vi "Graph ERD Read List_Brass.vi"(0 "GEA2 Reference In":refnum<k24>, 5 "GEA Inputs":T8={"Source"=229, "Destination"=50} {"Destination" format="%.0x"; "Source" format="%.0x"}, 7 "All_Bundled_Data_Brass":T1, 9 "ERD Graph Cntrl":T9={"ERD 3"={"ERD #"=0, "Data Type"=enum."uint16_t", "Scaler"=1}, "ERD 2"={"ERD #"=0, "Data Type"=enum."uint16_t", "Scaler"=1}, "ERD 1"={"ERD #"=0, "Data Type"=enum."uint16_t", "Scaler"=1}} {"ERD 1"."Scaler" min=1; "ERD 1"."ERD #" format="%.0x"; "ERD 2"."Scaler" min=1; "ERD 2"."ERD #" format="%.0x"; "ERD 3"."Scaler" min=1; "ERD 3"."ERD #" format="%.0x"}, 11 "Error In":errorcluster) -> (4 "GEA2 Reference Out":refnum<k24>, 6 "ERD Graph  Ind":T7, 10 "All_Bundled_Data_Brass 2":T1, 15 "Error Out":errorcluster)   [LabVIEW 2016]
uses:
  Laundry Tool 1.0 Support/type defs/ERD_Graph_All.ctl
  Laundry Tool 1.0 Support/type defs/ERD_Graph.ctl
  Common/LabVIEW GEA2 Toolkit/LabVIEW_GEA2_Toolkit.lvlibp/type defs/Data Type.ctl
  C:/Automation/DLLs/PC Dot Net/GeaCommunication.dll
  Common/LabVIEW GEA2 Toolkit/LabVIEW_GEA2_Toolkit.lvlibp/type defs/Source_Destination.ctl
  type defs2/All_Bundled_Data_Brass.ctl
  Laundry Tool 1.0 Support/type defs/Version.ctl
  type defs2/ERD_Always_Show_Brass.ctl
  type defs2/CSV_File_String_Arrays.ctl
  type defs2/Fault Table Array.ctl
  Laundry Tool 1.0 Support/type defs/Fault_Table_Info.ctl
  Common/LabVIEW GEA2 Toolkit/LabVIEW_GEA2_Toolkit.lvlibp/type defs/ERD Read Data In.ctl
  Common/LabVIEW GEA2 Toolkit/LabVIEW_GEA2_Toolkit.lvlibp
panel:
  # "Software Version"
  # "UI"
  # "MC"
  # "Software Version"
  # "UI"
  # "MC"
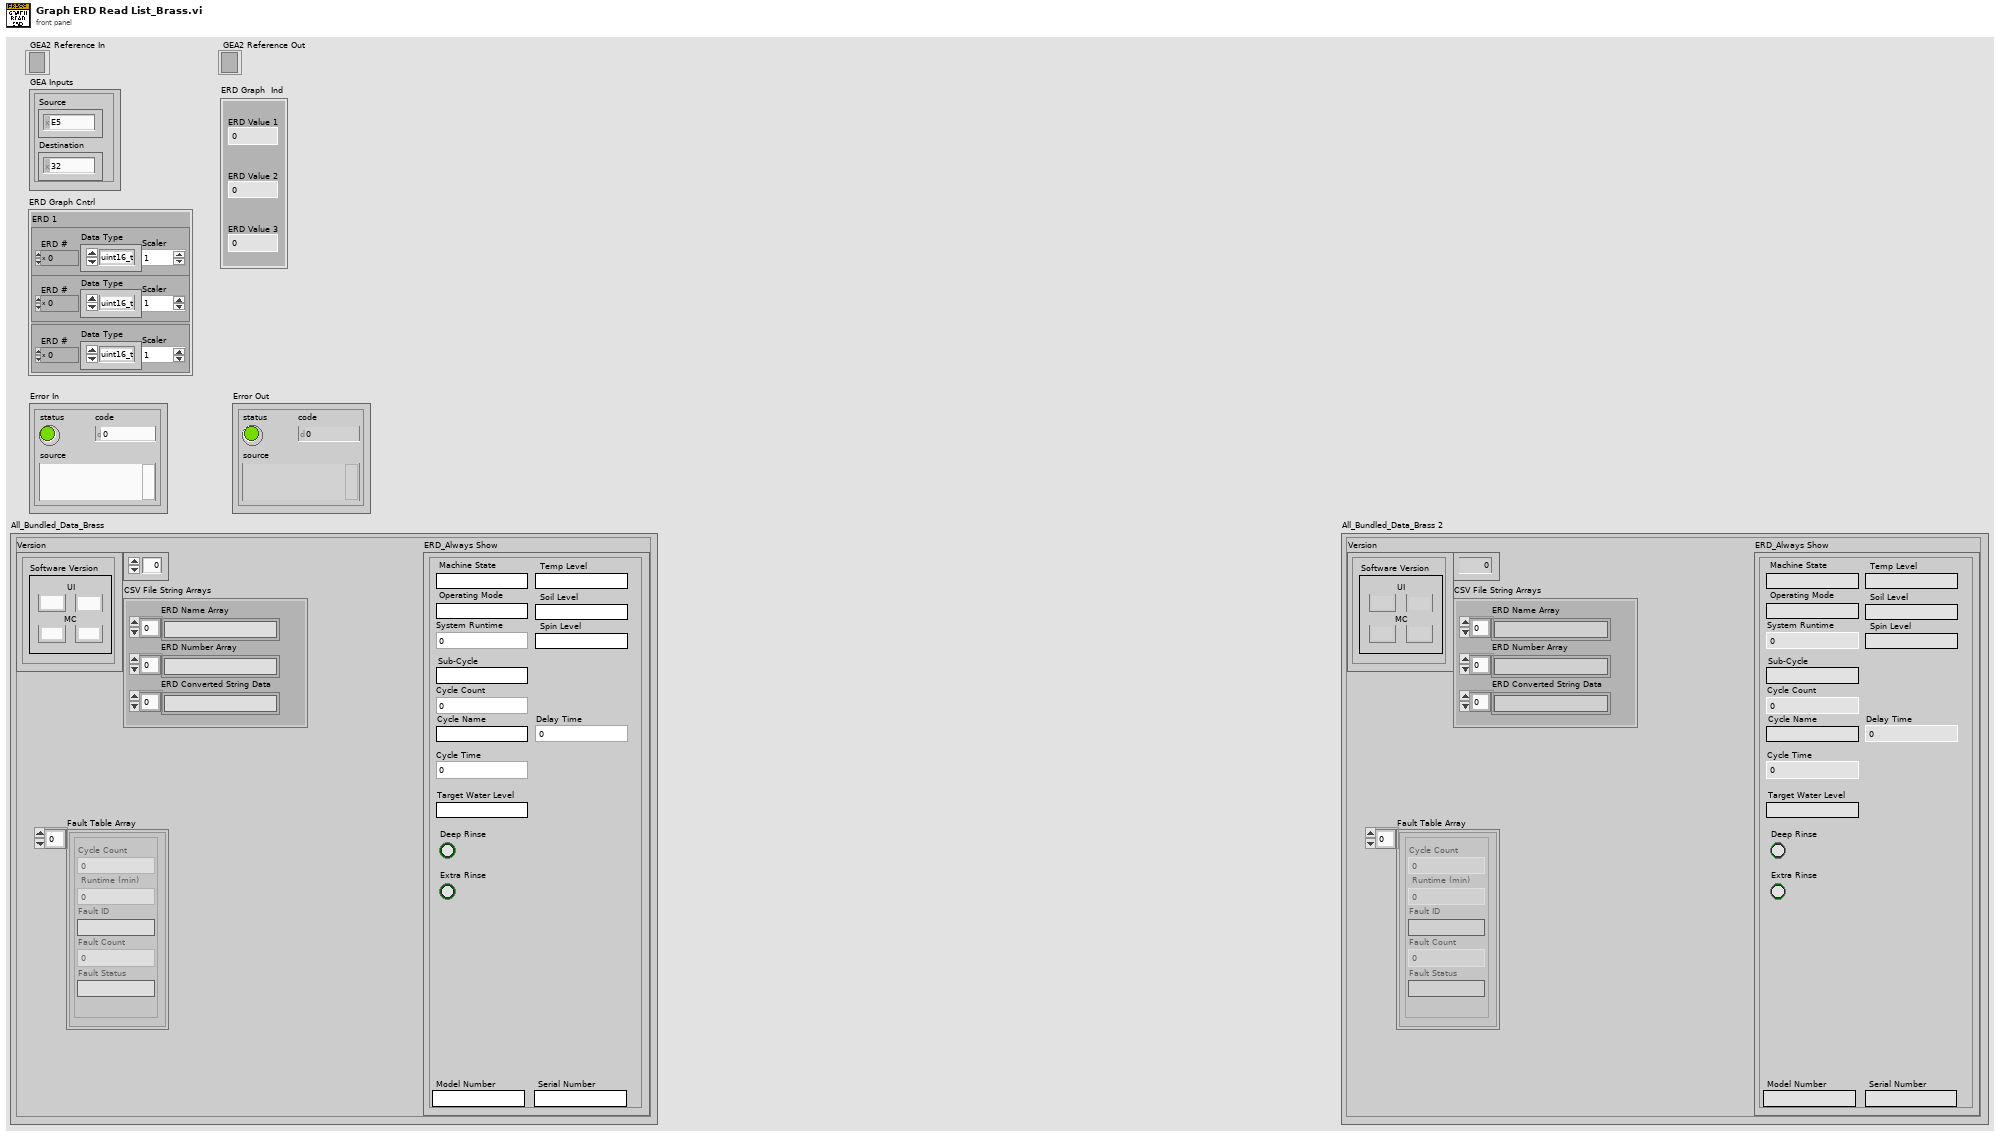
[diagram p1: front panel]
types:
  T1 = typedef "All_Bundled_Data_Brass.ctl" = cluster{"Version":T2, "ERD_Always Show":T3, "Personality Set":u8, "CSV File String Arrays":T4, "Fault Table Array ":T5}
  T2 = typedef "Version.ctl" = cluster{"Critical Major":string, "Critical Minor":string, "Non-Critical Minor":string, "Non-Critical Major":string}
  T3 = typedef "ERD_Always_Show_Brass.ctl" = cluster{"Machine State":string, "Cycle Count":u32, "Soil Level":string, "Spin Level":string, "Temp Level":string, "Delay Time":u16, "Sub-Cycle":string, "Cycle Name":string, "Model Number":string, "Serial Number":string, "System Runtime":u32, "Cycle Time":u16, "Operating Mode":string, "Target Water Level":string, "Deep Rinse":bool, "Extra Rinse":bool}
  T4 = typedef "CSV_File_String_Arrays.ctl" = cluster{"ERD Number Array":string[], "ERD Name Array":string[], "ERD Converted String Data":string[]}
  T5 = typedef "Fault Table Array.ctl" = T6[]
  T6 = typedef "Fault_Table_Info.ctl" = cluster{"Cycle Count":u32, " Runtime (min) ":u32, "Fault Status":string, "Fault ID":string, "Fault Count":u16}
  T7 = cluster{"ERD Value 1":dbl, "ERD Value 2":dbl, "ERD Value 3":dbl}
  T8 = typedef "LabVIEW_GEA2_Toolkit.lvlibp/Source_Destination.ctl" = cluster{"Source":u8, "Destination":u8}
  T9 = typedef "ERD_Graph_All.ctl" = cluster{"ERD 3":T10, "ERD 2":T10, "ERD 1":T10}
  T10 = typedef "ERD_Graph.ctl" = cluster{"ERD #":u16, "Data Type":T11, "Scaler":u32}
  T11 = typedef "LabVIEW_GEA2_Toolkit.lvlibp/Data Type.ctl" = enum16{"string", "boolean", "uint8_t", "uint16_t", "uint32_t", "uint64_t", "int8_t", "int16_t", "int32_t", "int64_t"}
  T12 = typedef "LabVIEW_GEA2_Toolkit.lvlibp/ERD Read Data In.ctl" = cluster{"ERD Number":u16, "Data Type":T11}
  T13 = typedef "LabVIEW_GEA2_Toolkit.lvlibp/ERD Read Data Out.ctl" = cluster{"ERD Number":u16, "Data":string}
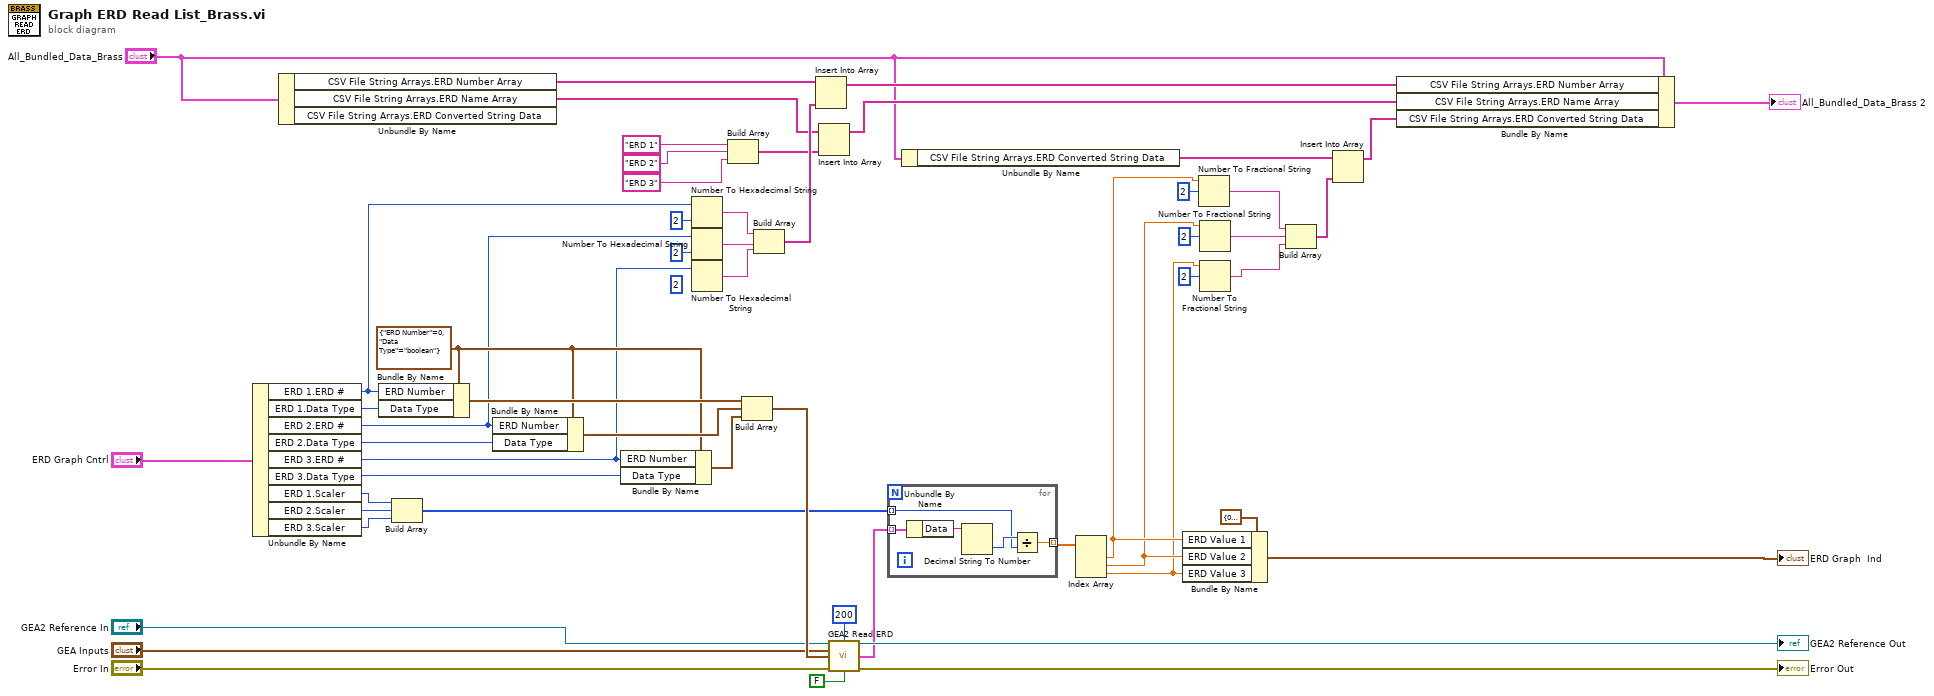
[diagram p0: block diagram]
diagram:
  (unwired) i16 2 ("width (-)")
  w51 = T12 {"ERD Number"=0, "Data Type"=enum."boolean"} ("ERD Read Data In 2")
  n1 = Unbundle By Name("ERD Graph Cntrl") -> ("ERD 1.ERD #"=w6:u16, "ERD 1.Data Type"=w48:T11, "ERD 2.ERD #"=w7:u16, "ERD 2.Data Type"=w49:T11, "ERD 3.ERD #"=w8:u16, "ERD 3.Data Type"=w50:T11, "ERD 1.Scaler"=w41:u32, "ERD 2.Scaler"=w40:u32, "ERD 3.Scaler"=w39:u32)
  n2 = Unbundle By Name("All_Bundled_Data_Brass") -> ("CSV File String Arrays.ERD Number Array"=w25:string[], "CSV File String Arrays.ERD Name Array"=w23:string[])  [unwired: 1 out]
  n3 = Bundle By Name(cluster=w51, "ERD Number"=w6, "Data Type"=w48) -> (w52:T12)
  n4 = Build Array(w41, w40, w39) -> (w38:u32[])
  n5 = Bundle By Name(cluster=w51, "ERD Number"=w7, "Data Type"=w49) -> (w53:T12)
  n6 = Bundle By Name(cluster=w51, "ERD Number"=w8, "Data Type"=w50) -> (w54:T12)
  n7 = Number To Hexadecimal String(1:i16 2 ("width (-)"), 2:w6) -> (0:w29:string)
  n8 = Number To Hexadecimal String(1:i16 2 ("width (-)"), 2:w7) -> (0:w28:string)
  n9 = Number To Hexadecimal String(2:w8) -> (0:w27:string)  [unwired: 1 in]
  n10 = Build Array("ERD 1", "ERD 2", "ERD 3") -> (w22:string[])
  n11 = Build Array(w52, w53, w54) -> (w47:T12[])
  n12 = Build Array(w29, w28, w27) -> (w26:string[])
  n13 = Insert Into Array(array=w25, new element=w26) -> (w24:string[])  [unwired: 1 in]
  n14 = Insert Into Array(array=w23, new element=w22) -> (w18:string[])  [unwired: 1 in]
  n15 = call "GEA2 Read ERD.vi"("GEA2 Reference In"="GEA2 Reference In", "Read Timeout (ms)"=u32 200, "GEA Inputs"="GEA Inputs", "Read ERD List"=w47, "Error In"="Error In", "Verify ERD Response?"=FALSE) -> ("GEA2 Reference Out"=→"GEA2 Reference Out":refnum<k24>, "ERD Data Out"=w37:T13[], "Error Out"=→"Error Out":errorcluster)  [unwired: 6 in, 1 out]
  n16 = for {
    tunnel: w38 -> [w57] mode=indexing
    tunnel: w37 -> [w60] mode=indexing
    tunnel: [w56] -> w36 mode=indexing
    n17 = Unbundle By Name(w60) -> ("Data"=w59:string)
    n18 = Decimal String To Number(string=w59) -> (number=w58:i32)  [unwired: 2 in, 1 out]
    n19 = Divide(x=w58, y=w57) -> (x/y=w56:dbl)
  }
  n20 = Unbundle By Name("All_Bundled_Data_Brass") -> ("CSV File String Arrays.ERD Converted String Data"=w11:string[])
  n21 = Index Array(array=w36) -> (element #1=w5:dbl, element #2=w4:dbl, element #3=w3:dbl)  [unwired: 3 in]
  n22 = Bundle By Name(cluster=T7 {"ERD Value 1"=0.0, "ERD Value 2"=0.0, "ERD Value 3"=0.0} ("ERD Graph  Ind"), "ERD Value 1"=w5, "ERD Value 2"=w4, "ERD Value 3"=w3) -> (→"ERD Graph  Ind":T7)
  n23 = Number To Fractional String(number=w5, width (-)=i16 2) -> (F-format string=w14:string)  [unwired: 2 in]
  n24 = Number To Fractional String(number=w4, width (-)=i16 2) -> (F-format string=w13:string)  [unwired: 2 in]
  n25 = Number To Fractional String(number=w3, width (-)=i16 2) -> (F-format string=w12:string)  [unwired: 2 in]
  n26 = Build Array(w14, w13, w12) -> (w10:string[])
  n27 = Insert Into Array(array=w11, new element=w10) -> (w9:string[])  [unwired: 1 in]
  n28 = Bundle By Name(cluster="All_Bundled_Data_Brass", "CSV File String Arrays.ERD Number Array"=w24, "CSV File String Arrays.ERD Name Array"=w18, "CSV File String Arrays.ERD Converted String Data"=w9) -> (→"All_Bundled_Data_Brass 2":T1)
